vi "main.vi"() -> ()   [LabVIEW 2015]
uses:
  <vilib>/Utility/NIReport.llb/NI_report.lvclass
  Agilent 3352X Series/Agilent 3352X Series.lvlib
  <vilib>/Utility/NIReport.llb/Excel/NI_Excel.lvclass
  <vilib>/addons/_office/NI_ReportGenerationToolkit.lvlib
  <vilib>/addons/_office/_exclsub.llb/font.ctl
panel:
  in  "退出":bool
  out "已连接":bool
  in  "连接设备":bool
  in  "原始记录模板":string(combo)="单向电荷型加速度传感器10-5000.xls"
  in  "出厂编号":string
  in  "被测通道":tag="PXI1Slot3/ai1" caption="标准通道"
  in  "方向选择":string(combo)="Z向"
  in  "参考通道":tag="PXI1Slot3/ai0" caption="标准通道"
  in  "信号发生器(33XXX系列)":refnum<visa-resource-name>="USB0::0x0957::0x2C07::MY52810975::INSTR"
  in  "保存":bool
  in  "停止":bool
  in  "测量":bool
  out "消息":string
  # "加速度传感器校准软件"
  # "仪器设置"
  # "参数配置"
  # "控制"
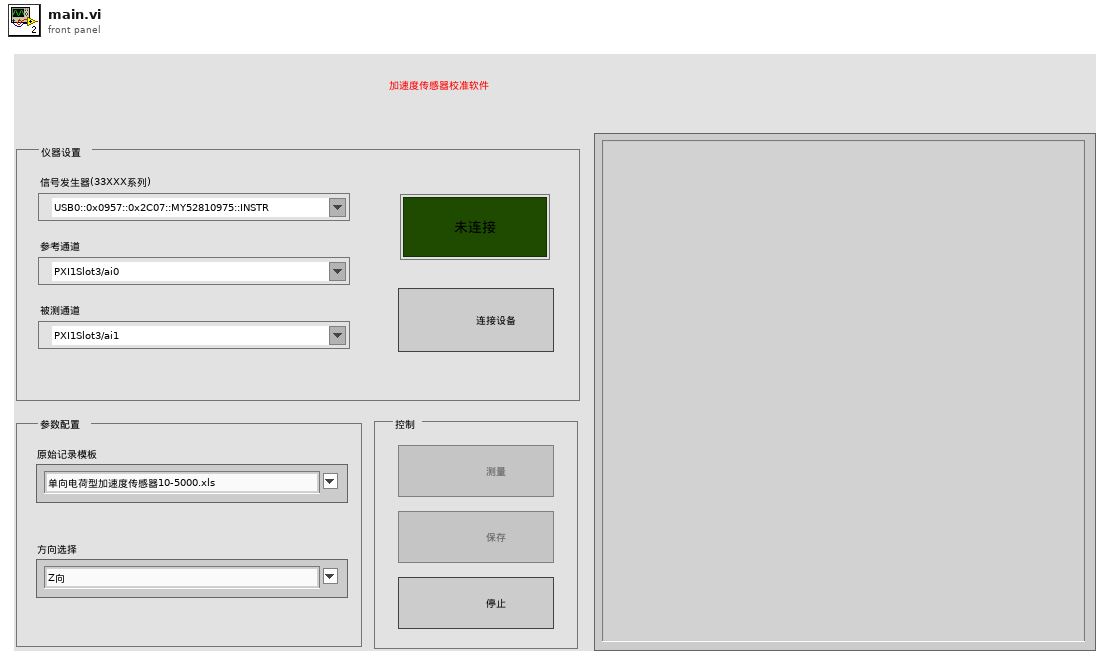
[diagram p1: front panel]
types:
  T1 = typedef "测试状态.ctl" = enum16{"idle", "路径配置", "参考灵敏度", "幅频响应", "幅值线性度", "结束", "停止"}
  T2 = typedef "句柄.ctl" = cluster{"33XXX":refnum<visa-resource-name>, "参考通道":tag, "被测通道":tag, "模板":refnum<class "NI_report.lvclass">}
  T3 = typedef "NI_ReportGenerationToolkit.lvlib/font.ctl" = cluster{"font name":string, "font size":dbl, "bold":u16, "italic":u16, "underline":u16, "strike through":u16, "font color":u32}
  T4 = enum16{"Standard Report", "HTML", "Word", "Excel"}
  T5 = enum16{"maximized", "minimized", "normal", "no change"}
  T6 = enum8{"Enabled", "Disabled", "Disabled and Grayed Out"}
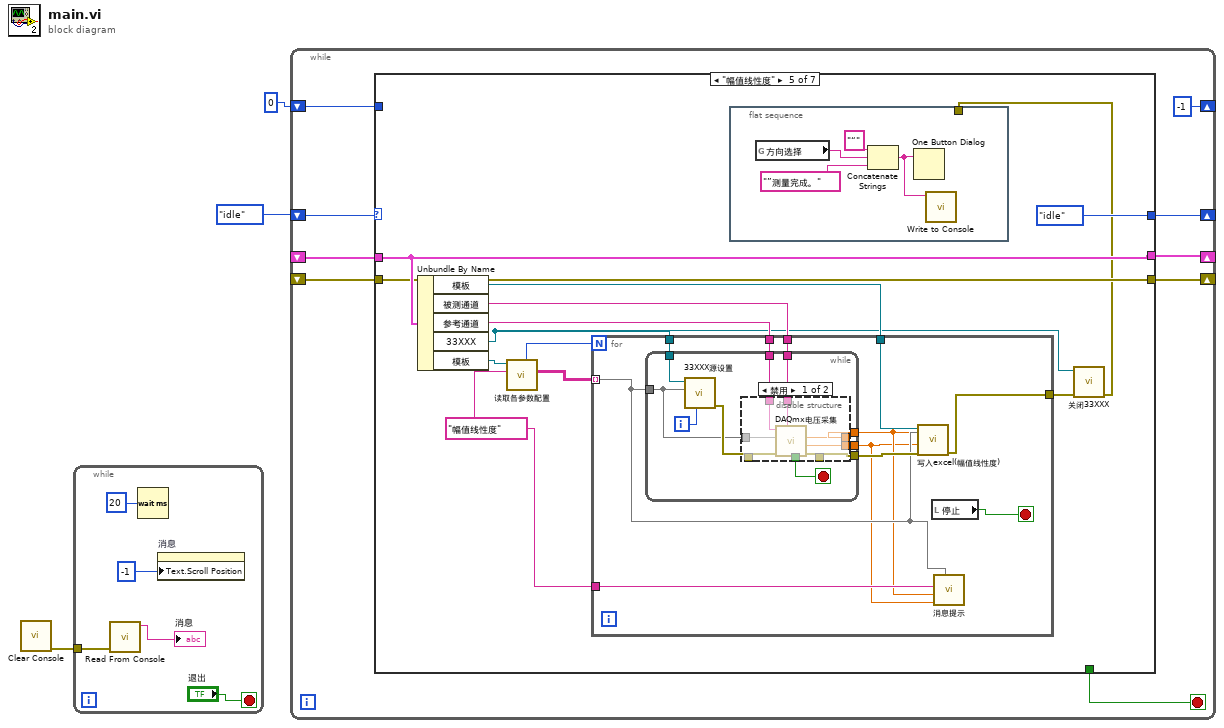
[diagram p0: block diagram]
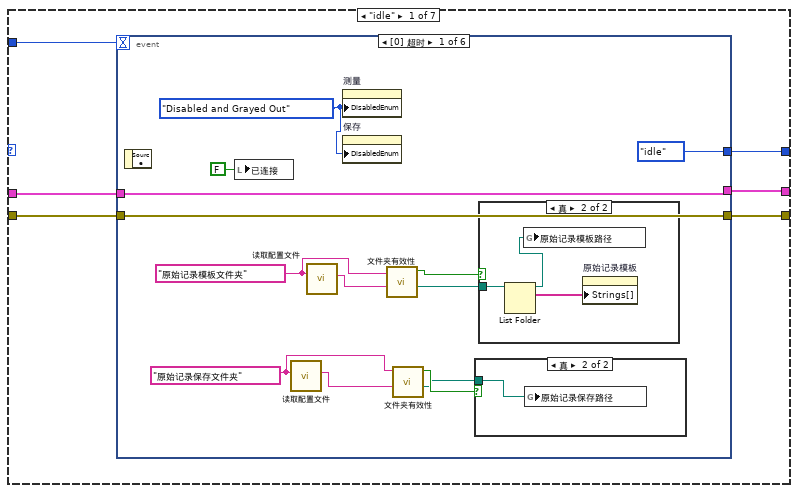
[diagram p2: hidden frame]
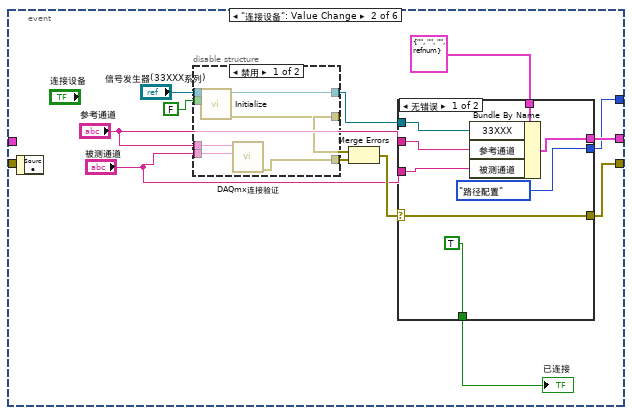
[diagram p5: hidden frame]
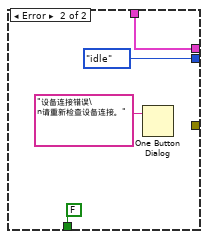
[diagram p7: hidden frame]
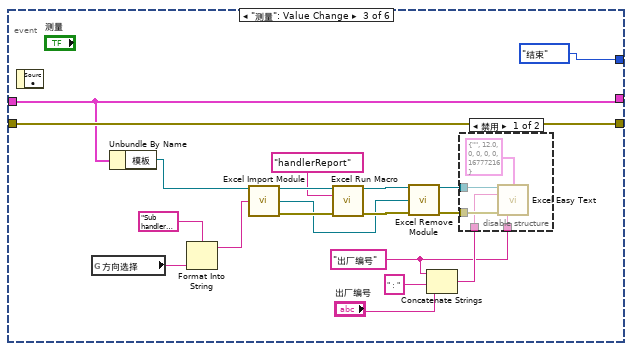
[diagram p8: hidden frame]
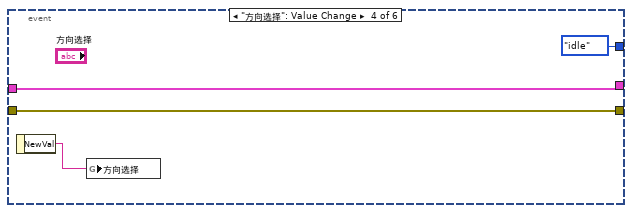
[diagram p10: hidden frame]
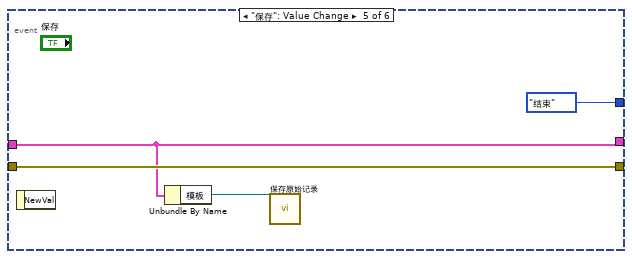
[diagram p11: hidden frame]
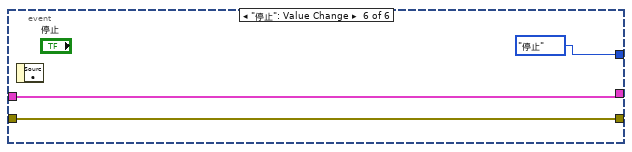
[diagram p12: hidden frame]
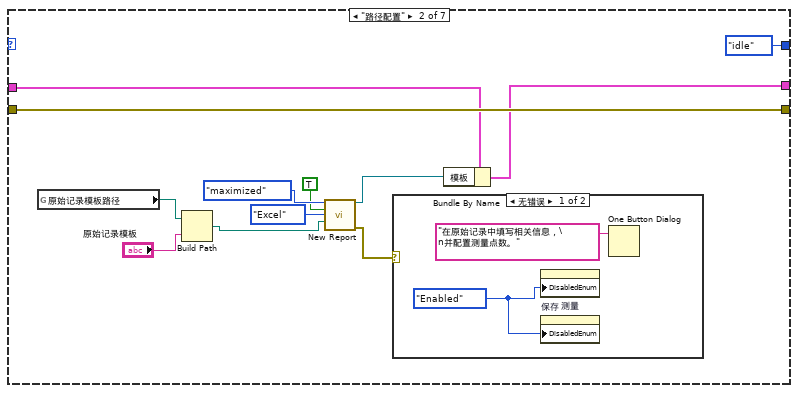
[diagram p13: hidden frame]
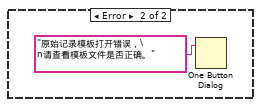
[diagram p14: hidden frame]
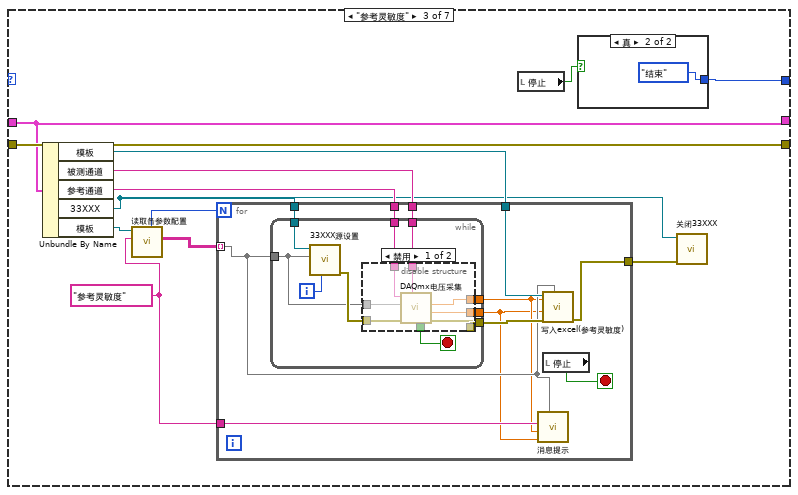
[diagram p15: hidden frame]
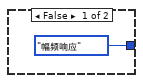
[diagram p16: hidden frame]
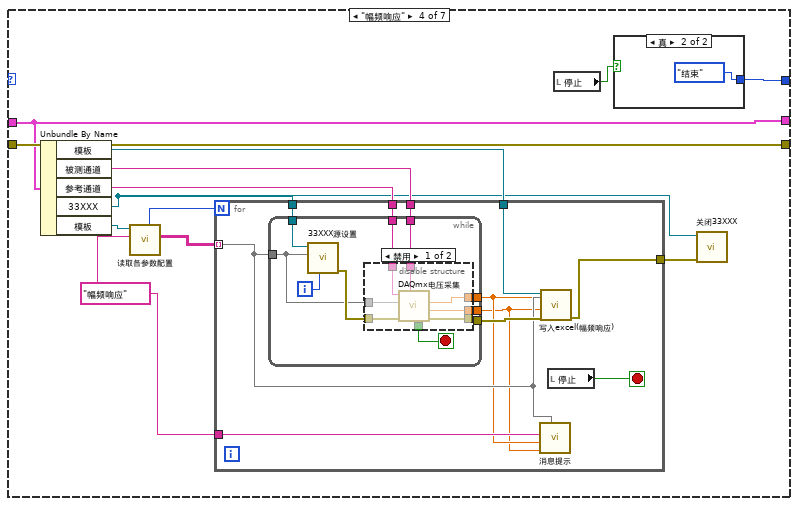
[diagram p18: hidden frame]
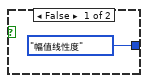
[diagram p19: hidden frame]
diagram:
  n1 = call "Clear Console.vi"() -> ("error out"=w1:errorcluster)  [unwired: 11 in]
  n2 = while {
    tunnel: w1 -> [w7]
    stop <- "退出" stop-if-true
    n3 = call "Read From Console.vi"("error in (no error)"=w7) -> ("Output"=→"消息":string)  [unwired: 9 in, 1 out]
    n4 = Wait (ms)(milliseconds to wait=u32 20) -> ()  [unwired: 1 out]
    n5 = property on="消息" class="Str"("Text.Scroll Position"=i8 -1 ("milliseconds to wait")) -> ()  [unwired: 2 in, 2 out]
  }
  n6 = while {
    shift-right: [w16] -> _
    shift-left: _ -> [w14]
    shift-right: [w15] -> _
    shift-left: _ -> [w13]
    shift-right: [w12] -> _
    shift-left: 测试状态."idle" ("枚举") -> [w17]
    shift-right: [-1] -> _
    shift-left: 0 -> [w10]
    stop <- w11 stop-if-true
    n7 = case shown="\"幅值线性度\"" w17 {
      tunnel: [w23 w109 w134 w169 w214 T2 {"33XXX"="", "参考通道"="", "被测通道"="", "模板"=refnum} T2 {"33XXX"="", "参考通道"="", "被测通道"="", "模板"=refnum}] -> w16
      tunnel: [w22 w118 w135 w170 w213 w257 w268] -> w15
      tunnel: w14 -> [w21 w111 w134 w169 w214 w262 _]
      tunnel: w13 -> [w20 w118 w135 w170 w213 w260 w268]
      tunnel: [w19 测试状态."idle" ("枚举") w124 w179 测试状态."idle" ("枚举") 测试状态."idle" ("枚举") 测试状态."idle" ("枚举")] -> w12
      tunnel: [_ _ _ _ _ FALSE TRUE] -> w11
      tunnel: w10 -> [w18 _ _ _ _ _ _]
      frame "idle" {
        n8 = event shown="[0] 超时" {
          selector: _ -> [_ _ _ _ _ _]
          dyn-events: _ -> [_ _ _ _ _ _]
          timeout: w18 -> [_ _ _ _ _ _]
          tunnel: [w36 w48 w89 w100 w102 w107] -> w23
          tunnel: [w35 w52 w91 w99 w104 w106] -> w22
          tunnel: w21 -> [w36 _ w89 w100 w102 w107]
          tunnel: w20 -> [w35 _ w91 w99 w104 w106]
          tunnel: [测试状态."idle" ("枚举") w41 测试状态."结束" ("枚举") 测试状态."idle" ("枚举") 测试状态."结束" ("枚举") 测试状态."停止" ("枚举")] -> w19
          event Timeout {
            w24 = T6."Disabled and Grayed Out" ("禁用")
            w27 = "原始记录保存文件夹" ("配置")
            w32 = "原始记录模板文件夹" ("配置")
            n9 = event-data() -> ()  [unwired: 1 in, 1 out]
            n10 = local write "已连接"(FALSE ("已连接")) -> ()
            n11 = call "读取配置文件.vi"("配置"=w27) -> ("路径"=w28:string)  [unwired: 9 in, 1 out]
            n12 = call "读取配置文件.vi"("配置"=w32) -> ("路径"=w31:string)  [unwired: 9 in, 1 out]
            n13 = property on="测量" class="Bool"("DisabledEnum"=w24) -> ()  [unwired: 2 in, 2 out]
            n14 = property on="保存" class="Bool"("DisabledEnum"=w24) -> ()  [unwired: 2 in, 2 out]
            n15 = call "文件夹有效性.vi"("路径"=w31, "配置"=w32) -> ("路径"=w30:path, "Valid"=w29:bool)  [unwired: 8 in]
            n16 = call "文件夹有效性.vi"("路径"=w28, "配置"=w27) -> ("路径"=w25:path, "Valid"=w26:bool)  [unwired: 8 in]
            n17 = case shown="真" w26 {
              tunnel: w25 -> [_ w37]
              frame False {
              }
              frame True {
                n18 = global write "Global.vi" "原始记录保存路径"(w37) -> ()
              }
            }
            n19 = case shown="真" w29 {
              tunnel: w30 -> [_ w40]
              frame False {
              }
              frame True {
                n20 = List Folder(path=w40) -> (path out=w38:path, filenames=w39:string[])  [unwired: 3 in, 2 out]
                n21 = global write "Global.vi" "原始记录模板路径"(w38) -> ()
                n22 = property on="原始记录模板" class="CmbBox"("Strings[]"=w39) -> ()  [unwired: 2 in, 2 out]
              }
            }
          }
          event "连接设备": Value Change {
            n23 = event-data() -> ()  [unwired: 1 in, 1 out]
            n24 = disable-structure shown="禁用" {
              disable-tunnel: [w60 _] -> w50
              disable-tunnel: "参考通道" -> [w59 _]
              disable-tunnel: "被测通道" -> [w58 _]
              disable-tunnel: "信号发生器(33XXX系列)" -> [w57 _]
              disable-tunnel: FALSE ("ID Query (True)") -> [w56 _]
              disable-tunnel: [w55 _] -> w43
              disable-tunnel: [w54 _] -> w42
              frame Disabled {
                n25 = call "Initialize.vi"("ID Query (Enable)"=w56, "VISA resource name"=w57) -> ("error out"=w54:errorcluster, "VISA resource name out"=w55:refnum<visa-resource-name>)  [unwired: 8 in]
                n26 = call "DAQmx连接验证.vi"("被测"=w58, "参考"=w59) -> ("error out"=w60:errorcluster)  [unwired: 9 in]
              }
              frame Enabled {
              }
            }
            n27 = Merge Errors(w42, w50) -> (w53:errorcluster)
            n28 = case shown="无错误" w53 {
              selector: w53 -> [w67 _]
              tunnel: w43 -> [w68 _]
              tunnel: "参考通道" -> [w65 _]
              tunnel: [w64 w70] -> w48
              tunnel: [w67 _] -> w52
              tunnel: [TRUE FALSE ("已连接")] -> w51
              tunnel: "被测通道" -> [w63 _]
              tunnel: T2 {"33XXX"="", "参考通道"="", "被测通道"="", "模板"=refnum} -> [w62 w70]
              tunnel: [测试状态."路径配置" ("枚举") 测试状态."idle" ("枚举")] -> w41
              frame No Error {
                n29 = Bundle By Name(cluster=w62, "33XXX"=w68, "参考通道"=w65, "被测通道"=w63) -> (w64:T2)
              }
              frame Error {
                n30 = One Button Dialog(message="设备连接错误\n请重新检查设备连接。") -> ()  [unwired: 1 in, 1 out]
              }
            }
            "已连接" <- w51
          }
          event "测量": Value Change {
            w74 = "出厂编号"
            n31 = event-data() -> ()  [unwired: 1 in, 1 out]
            n32 = global read "Global.vi" "方向选择"() -> (w81:string)
            n33 = Unbundle By Name(w89) -> ("模板"=w88:refnum<class "NI_report.lvclass">)
            n34 = Format Into String(format string="Sub handlerReport()\n    Dim count As Integer\n    Dim col As String\n    Dim cuRange As String\n    Sheets(\"%S\").Select\n    '幅频响应\n    count = Sheets(\"测量点数\").Range(\"B2\")\n    If count <= 6 Then\n        Rows(\"16:27\").Hidden = True\n        col = CNtoW(count + 2)\n        cuRange = col & (10) & \":H\" & (15)\n        Range(cuRange).ClearContents\n    ElseIf count <= 12 Then\n        Rows(\"22:27\").Hidden = True\n        col = CNtoW(count - 6 + 2)\n        cuRange = col & (16) & \":H\" & (21)\n        Range(cuRange).ClearContents\n    ElseIf count <= 16 Then\n        col = CNtoW(count - 12 + 2)\n        cuRange = col & (22) & \":H\" & (27)\n        Range(cuRange).ClearContents\n    Else\n    End If\n    Call hideAmpborder(count, cuRange)\n    '幅值线性度\n    count = Sheets(\"测量点数\").Range(\"B3\")\n    If count <= 5 Then\n        Rows(\"35:40\").Hidden = True\n        col = CNtoW(count + 2)\n        cuRange = col & (29) & \":H\" & (34)\n        Range(cuRange).ClearContents\n    ElseIf count <= 10 Then\n        col = CNtoW(count - 5 + 2)\n        cuRange = col & (35) & \":H\" & (40)\n        Range(cuRange).ClearContents\n    Else\n    End If\n    Call hideLineborder(count, cuRange)\nEnd Sub\n'列数转字母\nFunction CNtoW(ByVal num As Long) As String\n    CNtoW = Replace(Cells(1, num).Address(False, False), \"1\", \"\")\nEnd Function\n'隐藏边框(幅频响应)\nFunction hideAmpborder(ByVal hideCount As Integer, ByVal hideRange As String)\n    If hideCount <= 6 Then\n        Range(hideRange).Select\n        Selection.Borders(xlEdgeTop).LineStyle = xlNone\n        Selection.Borders(xlEdgeBottom).LineStyle = xlNone\n        Selection.Borders(xlEdgeRight).LineStyle = xlNone\n        Selection.Borders(xlInsideVertical).LineStyle = xlNone\n        Selection.Borders(xlInsideHorizontal).LineStyle = xlNone\n    ElseIf hideCount <= 16 Then\n        Range(hideRange).Select\n        Selection.Borders(xlEdgeBottom).LineStyle = xlNone\n        Selection.Borders(xlEdgeRight).LineStyle = xlNone\n        Selection.Borders(xlInsideVertical).LineStyle = xlNone\n        Selection.Borders(xlInsideHorizontal).LineStyle = xlNone\n    End If\nEnd Function\n'隐藏边框(幅值线性度)\nFunction hideLineborder(ByVal hideCount As Integer, ByVal hideRange As String)\n    If hideCount <= 5 Then\n        Range(hideRange).Select\n        Selection.Borders(xlEdgeTop).LineStyle = xlNone\n        Selection.Borders(xlEdgeBottom).LineStyle = xlNone\n        Selection.Borders(xlEdgeRight).LineStyle = xlNone\n        Selection.Borders(xlInsideVertical).LineStyle = xlNone\n        Selection.Borders(xlInsideHorizontal).LineStyle = xlNone\n    ElseIf hideCount <= 10 Then\n        Range(hideRange).Select\n        Selection.Borders(xlEdgeBottom).LineStyle = xlNone\n        Selection.Borders(xlEdgeRight).LineStyle = xlNone\n        Selection.Borders(xlInsideVertical).LineStyle = xlNone\n        Selection.Borders(xlInsideHorizontal).LineStyle = xlNone\n    End If\nEnd Function", w81) -> (resulting string=w80:string)  [unwired: 2 in, 1 out]
            n35 = call <vilib>:"Excel Import Module.vi"("report in"=w88, "module code (\"\")"=w80) -> ("report out"=w87:refnum<class "NI_report.lvclass">, "module reference"=w82:refnum<k7>, "error out"=w86:errorcluster)  [unwired: 11 in]
            n36 = call <vilib>:"Excel Run Macro.vi"("report in"=w87, "macro name"="handlerReport", "error in (no error)"=w86) -> ("report out"=w84:refnum<class "NI_report.lvclass">, "error out"=w83:errorcluster)  [unwired: 10 in, 1 out]
            n37 = call <vilib>:"Excel Remove Module.vi"("report in"=w84, "module reference"=w82, "error in (no error)"=w83) -> ("report out"=w79:refnum<class "NI_report.lvclass">, "error out"=w78:errorcluster)  [unwired: 11 in]
            n38 = Concatenate Strings(w74, "：", "出厂编号") -> (w76:string)
            n39 = disable-structure shown="禁用" {
              disable-tunnel: w79 -> [w96 _]
              disable-tunnel: w78 -> [w95 _]
              disable-tunnel: w76 -> [w94 _]
              disable-tunnel: w74 -> [w93 _]
              frame Disabled {
                n40 = call <vilib>:"Excel Easy Text.vi"("report in"=w96, "font"=T3 {"font name"="", "font size"=12.0, "bold"=0, "italic"=0, "underline"=0, "strike through"=0, "font color"=16777216}, "text"=w94, "error in (no error)"=w95, "name (\"\")"=w93) -> ()  [unwired: 6 in, 5 out]
              }
              frame Enabled {
              }
            }
          }
          event "方向选择": Value Change {
            n41 = event-data() -> ("NewVal"=w97:string)  [unwired: 1 in]
            n42 = global write "Global.vi" "方向选择"(w97) -> ()
          }
          event "保存": Value Change {
            n43 = event-data() -> ()  [unwired: 1 in, 1 out]
            n44 = Unbundle By Name(w102) -> ("模板"=w101:refnum<class "NI_report.lvclass">)
            n45 = call "保存原始记录.vi"("NI_report输入"=w101) -> ()  [unwired: 10 in, 1 out]
          }
          event "停止": Value Change {
            n46 = event-data() -> ()  [unwired: 1 in, 1 out]
          }
        }
      }
      frame "路径配置" {
        n47 = global read "Global.vi" "原始记录模板路径"() -> (w117:path)
        n48 = Build Path(base path=w117, name or relative path="原始记录模板") -> (appended path=w112:path)
        n49 = call <vilib>:"New Report.vi"("window state (normal)"=T5."maximized", "display alerts? (F)"=TRUE, "report type"=T4."Excel", "template (empty)"=w112) -> ("report out"=w110:refnum<class "NI_report.lvclass">, "error out"=w108:errorcluster)  [unwired: 10 in]
        n50 = case shown="无错误" w108 {
          frame No Error {
            w120 = T6."Enabled" ("禁用")
            n51 = property on="测量" class="Bool"("DisabledEnum"=w120) -> ()  [unwired: 2 in, 2 out]
            n52 = property on="保存" class="Bool"("DisabledEnum"=w120) -> ()  [unwired: 2 in, 2 out]
            n53 = One Button Dialog(message="在原始记录中填写相关信息，\n并配置测量点数。" ("消息")) -> ()  [unwired: 1 in, 1 out]
          }
          frame Error {
            n54 = One Button Dialog(message="原始记录模板打开错误，\n请查看模板文件是否正确。" ("消息")) -> ()  [unwired: 1 in, 1 out]
          }
        }
        n55 = Bundle By Name(cluster=w111, "模板"=w110) -> (w109:T2)
      }
      frame "参考灵敏度" {
        w123 = "参考灵敏度" ("参数")
        n56 = Unbundle By Name(w134) -> ("模板"=w128:refnum<class "NI_report.lvclass">, "被测通道"=w130:tag, "参考通道"=w129:tag, "33XXX"=w126:refnum<visa-resource-name>, "模板"=w133:refnum<class "NI_report.lvclass">)
        n57 = call "读取各参数配置.vi"("参数"=w123, "NI_report输入"=w133) -> ("设置"=w131:string[][], "测量点数"=w132:i32)  [unwired: 6 in, 2 out]
        n58 = for {
          N: w132 -> [_]
          tunnel: w131 -> [w141] mode=indexing
          tunnel: w126 -> [w148]
          tunnel: w130 -> [w147]
          tunnel: w129 -> [w146]
          tunnel: w128 -> [w145]
          tunnel: [w143] -> w127
          tunnel: w123 -> [w140]
          stop <- w142 stop-if-true
          n59 = while {
            tunnel: w141 -> [w153]
            tunnel: w148 -> [w157]
            tunnel: w147 -> [w156]
            tunnel: w146 -> [w155]
            tunnel: [w151] -> w139
            tunnel: [w150] -> w138
            tunnel: [w149] -> w144
            i -> [w158]
            stop <- w152 stop-if-true
            n60 = call "33XXX源设置.vi"("步长"=w158, "设置"=w153, "VISA引用句柄输入"=w157) -> ("error out"=w154:errorcluster)  [unwired: 7 in, 1 out]
            n61 = disable-structure shown="禁用" {
              disable-tunnel: w156 -> [w166 _]
              disable-tunnel: w155 -> [w165 _]
              disable-tunnel: w154 -> [w164 _]
              disable-tunnel: w153 -> [w163 _]
              disable-tunnel: [w162 _] -> w152
              disable-tunnel: [w161 _] -> w151
              disable-tunnel: [w160 _] -> w150
              disable-tunnel: [w159 _] -> w149
              frame Disabled {
                n62 = call "DAQmx电压采集.vi"("被测通道"=w166, "error in"=w164, "设置"=w163, "参考通道"=w165) -> ("error out"=w159:errorcluster, "被测幅值"=w160:dbl, "参考幅值"=w161:dbl, "满足条件"=w162:bool)  [unwired: 4 in]
              }
              frame Enabled {
              }
            }
          }
          n63 = call "消息提示.vi"("设置"=w141, "被测幅值"=w138, "参考幅值"=w139, "参数"=w140) -> ()  [unwired: 8 in]
          n64 = call "写入excel(参考灵敏度).vi"("设置"=w141, "error in (no error)"=w144, "被测幅值"=w138, "参考幅值"=w139, "NI_report输入"=w145) -> ("error out"=w143:errorcluster)  [unwired: 5 in, 1 out]
          n65 = local read "停止"() -> (w142:bool)
        }
        n66 = local read "停止"() -> (w125:bool)
        n67 = case shown="真" w125 {
          tunnel: [测试状态."幅频响应" ("枚举") 测试状态."结束" ("枚举")] -> w124
          frame False {
          }
          frame True {
          }
        }
        n68 = call "关闭33XXX.vi"("error in"=w127, "VISA引用句柄输入"=w126) -> ()  [unwired: 8 in, 2 out]
      }
      frame "幅频响应" {
        w167 = "幅频响应" ("参数")
        n69 = Unbundle By Name(w169) -> ("模板"=w173:refnum<class "NI_report.lvclass">, "被测通道"=w175:tag, "参考通道"=w174:tag, "33XXX"=w171:refnum<visa-resource-name>, "模板"=w178:refnum<class "NI_report.lvclass">)
        n70 = call "读取各参数配置.vi"("参数"=w167, "NI_report输入"=w178) -> ("设置"=w176:string[][], "测量点数"=w177:i32)  [unwired: 6 in, 2 out]
        n71 = for {
          N: w177 -> [_]
          tunnel: w176 -> [w185] mode=indexing
          tunnel: w171 -> [w192]
          tunnel: w175 -> [w191]
          tunnel: w174 -> [w190]
          tunnel: w173 -> [w189]
          tunnel: [w187] -> w172
          tunnel: w167 -> [w184]
          stop <- w186 stop-if-true
          n72 = while {
            tunnel: w185 -> [w197]
            tunnel: w192 -> [w201]
            tunnel: w191 -> [w200]
            tunnel: w190 -> [w199]
            tunnel: [w195] -> w183
            tunnel: [w194] -> w182
            tunnel: [w193] -> w188
            i -> [w202]
            stop <- w196 stop-if-true
            n73 = call "33XXX源设置.vi"("步长"=w202, "设置"=w197, "VISA引用句柄输入"=w201) -> ("error out"=w198:errorcluster)  [unwired: 7 in, 1 out]
            n74 = disable-structure shown="禁用" {
              disable-tunnel: w200 -> [w210 _]
              disable-tunnel: w199 -> [w209 _]
              disable-tunnel: w198 -> [w208 _]
              disable-tunnel: w197 -> [w207 _]
              disable-tunnel: [w206 _] -> w196
              disable-tunnel: [w205 _] -> w195
              disable-tunnel: [w204 _] -> w194
              disable-tunnel: [w203 _] -> w193
              frame Disabled {
                n75 = call "DAQmx电压采集.vi"("被测通道"=w210, "error in"=w208, "设置"=w207, "参考通道"=w209) -> ("error out"=w203:errorcluster, "被测幅值"=w204:dbl, "参考幅值"=w205:dbl, "满足条件"=w206:bool)  [unwired: 4 in]
              }
              frame Enabled {
              }
            }
          }
          n76 = call "消息提示.vi"("设置"=w185, "被测幅值"=w182, "参考幅值"=w183, "参数"=w184) -> ()  [unwired: 8 in]
          n77 = call "写入excel(幅频响应).vi"("设置"=w185, "error in (no error)"=w188, "被测幅值"=w182, "参考幅值"=w183, "NI_report输入"=w189) -> ("error out"=w187:errorcluster)  [unwired: 5 in, 1 out]
          n78 = local read "停止"() -> (w186:bool)
        }
        n79 = local read "停止"() -> (w168:bool)
        n80 = case shown="真" w168 {
          tunnel: [测试状态."幅值线性度" ("枚举") 测试状态."结束" ("枚举")] -> w179
          frame False {
          }
          frame True {
          }
        }
        n81 = call "关闭33XXX.vi"("error in"=w172, "VISA引用句柄输入"=w171) -> ()  [unwired: 8 in, 2 out]
      }
      frame "幅值线性度" {
        w211 = "幅值线性度" ("参数")
        n82 = Unbundle By Name(w214) -> ("模板"=w217:refnum<class "NI_report.lvclass">, "被测通道"=w219:tag, "参考通道"=w218:tag, "33XXX"=w215:refnum<visa-resource-name>, "模板"=w222:refnum<class "NI_report.lvclass">)
        n83 = call "读取各参数配置.vi"("参数"=w211, "NI_report输入"=w222) -> ("设置"=w220:string[][], "测量点数"=w221:i32)  [unwired: 6 in, 2 out]
        n84 = for {
          N: w221 -> [_]
          tunnel: w220 -> [w231] mode=indexing
          tunnel: w215 -> [w238]
          tunnel: w219 -> [w237]
          tunnel: w218 -> [w236]
          tunnel: w217 -> [w235]
          tunnel: [w233] -> w216
          tunnel: w211 -> [w230]
          stop <- w232 stop-if-true
          n85 = while {
            tunnel: w231 -> [w243]
            tunnel: w238 -> [w247]
            tunnel: w237 -> [w246]
            tunnel: w236 -> [w245]
            tunnel: [w241] -> w229
            tunnel: [w240] -> w228
            tunnel: [w239] -> w234
            i -> [w248]
            stop <- w242 stop-if-true
            n86 = call "33XXX源设置.vi"("步长"=w248, "设置"=w243, "VISA引用句柄输入"=w247) -> ("error out"=w244:errorcluster)  [unwired: 7 in, 1 out]
            n87 = disable-structure shown="禁用" {
              disable-tunnel: w246 -> [w256 _]
              disable-tunnel: w245 -> [w255 _]
              disable-tunnel: w244 -> [w254 _]
              disable-tunnel: w243 -> [w253 _]
              disable-tunnel: [w252 _] -> w242
              disable-tunnel: [w251 _] -> w241
              disable-tunnel: [w250 _] -> w240
              disable-tunnel: [w249 _] -> w239
              frame Disabled {
                n88 = call "DAQmx电压采集.vi"("被测通道"=w256, "error in"=w254, "设置"=w253, "参考通道"=w255) -> ("error out"=w249:errorcluster, "被测幅值"=w250:dbl, "参考幅值"=w251:dbl, "满足条件"=w252:bool)  [unwired: 4 in]
              }
              frame Enabled {
              }
            }
          }
          n89 = call "写入excel(幅值线性度).vi"("设置"=w231, "error in (no error)"=w234, "被测幅值"=w228, "参考幅值"=w229, "NI_report输入"=w235) -> ("error out"=w233:errorcluster)  [unwired: 5 in, 1 out]
          n90 = local read "停止"() -> (w232:bool)
          n91 = call "消息提示.vi"("设置"=w231, "被测幅值"=w228, "参考幅值"=w229, "参数"=w230) -> ()  [unwired: 8 in]
        }
        n92 = flat-sequence {
          tunnel: w212 -> [_]
          frame #0 {
            n93 = global read "Global.vi" "方向选择"() -> (w227:string)
            n94 = Concatenate Strings("“" ("字符串"), w227, "”测量完成。" ("字符串")) -> (w224:string)
            n95 = One Button Dialog(message=w224) -> ()  [unwired: 1 in, 1 out]
            n96 = call "Write to Console.vi"("Input"=w224) -> ()  [unwired: 10 in, 1 out]
          }
        }
        n97 = call "关闭33XXX.vi"("error in"=w216, "VISA引用句柄输入"=w215) -> ("error out"=w212:errorcluster)  [unwired: 8 in, 1 out]
      }
      frame "结束" {
        n98 = Unbundle By Name(w262) -> ("33XXX"=w261:refnum<visa-resource-name>)
        n99 = local write "已连接"(FALSE ("已连接")) -> ()
        n100 = disable-structure shown="禁用" {
          disable-tunnel: w261 -> [w267 _]
          disable-tunnel: w260 -> [w266 _]
          disable-tunnel: [w265 _] -> w257
          frame Disabled {
            n101 = call "Close.vi"("error in (no error)"=w266, "VISA resource name"=w267) -> ("error out"=w265:errorcluster)  [unwired: 9 in]
          }
          frame Enabled {
          }
        }
      }
      frame "停止" {
      }
    }
  }
